vi "GOOP_TcpIpListener.vi"() -> ()   [LabVIEW 2020]
uses:
  <resource>/Framework/Providers/Open_GDS/SubVIs/GOOP_UMLEditor_CallMainAction.ctl
panel:
  out "error out":errorcluster
  out "Numeric 2":u32
  out "remote port":u16
  out "remote address":string
  out "Numeric":i32
  out "data out":string
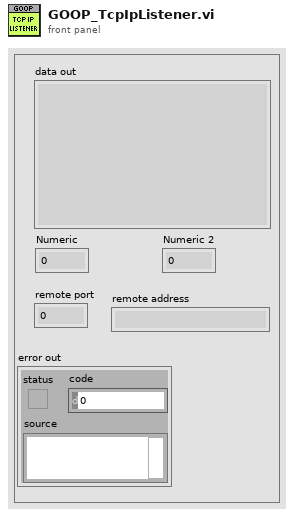
[diagram p1: front panel]
types:
  T1 = enum32{"invalid OS target", "Mac OS", "Windows 3.1", "Windows 95/NT", "Solaris 1", "Solaris 2", "HP-UX", "PowerMAX", "Linux", "Irix", "Rhapsody", "BeOS", "AIX", "OSF1", "VxWorks", "PharLap", "Carbon", "RTX", "Windows x64", "Linux x64"}
  T2 = enum32{"invalid OS target", "Mac OS", "Windows 3.1", "Windows 95/NT", "Solaris 1", "Solaris 2", "HP-UX", "PowerMAX", "Linux", "Irix", "Rhapsody", "BeOS", "AIX", "OSF1", "VxWorks", "PharLap", "Carbon", "RTX", "Windows x64", "Linux x64", "Mac OS X x64"}
  T3 = enum16{"Standard", "Buffered", "CRLF", "Immediate"}
  T4 = typedef "GOOP_UMLEditor_CallMainAction.ctl" = enum16{"OpenUmlEditor", "ReverseEngineering:WholeProject", "ReverseEngineering:OneClass", "ReverseEngineering:OneVI", "ShowInStateDiagram:OneVI", "OpenUMLFile"}
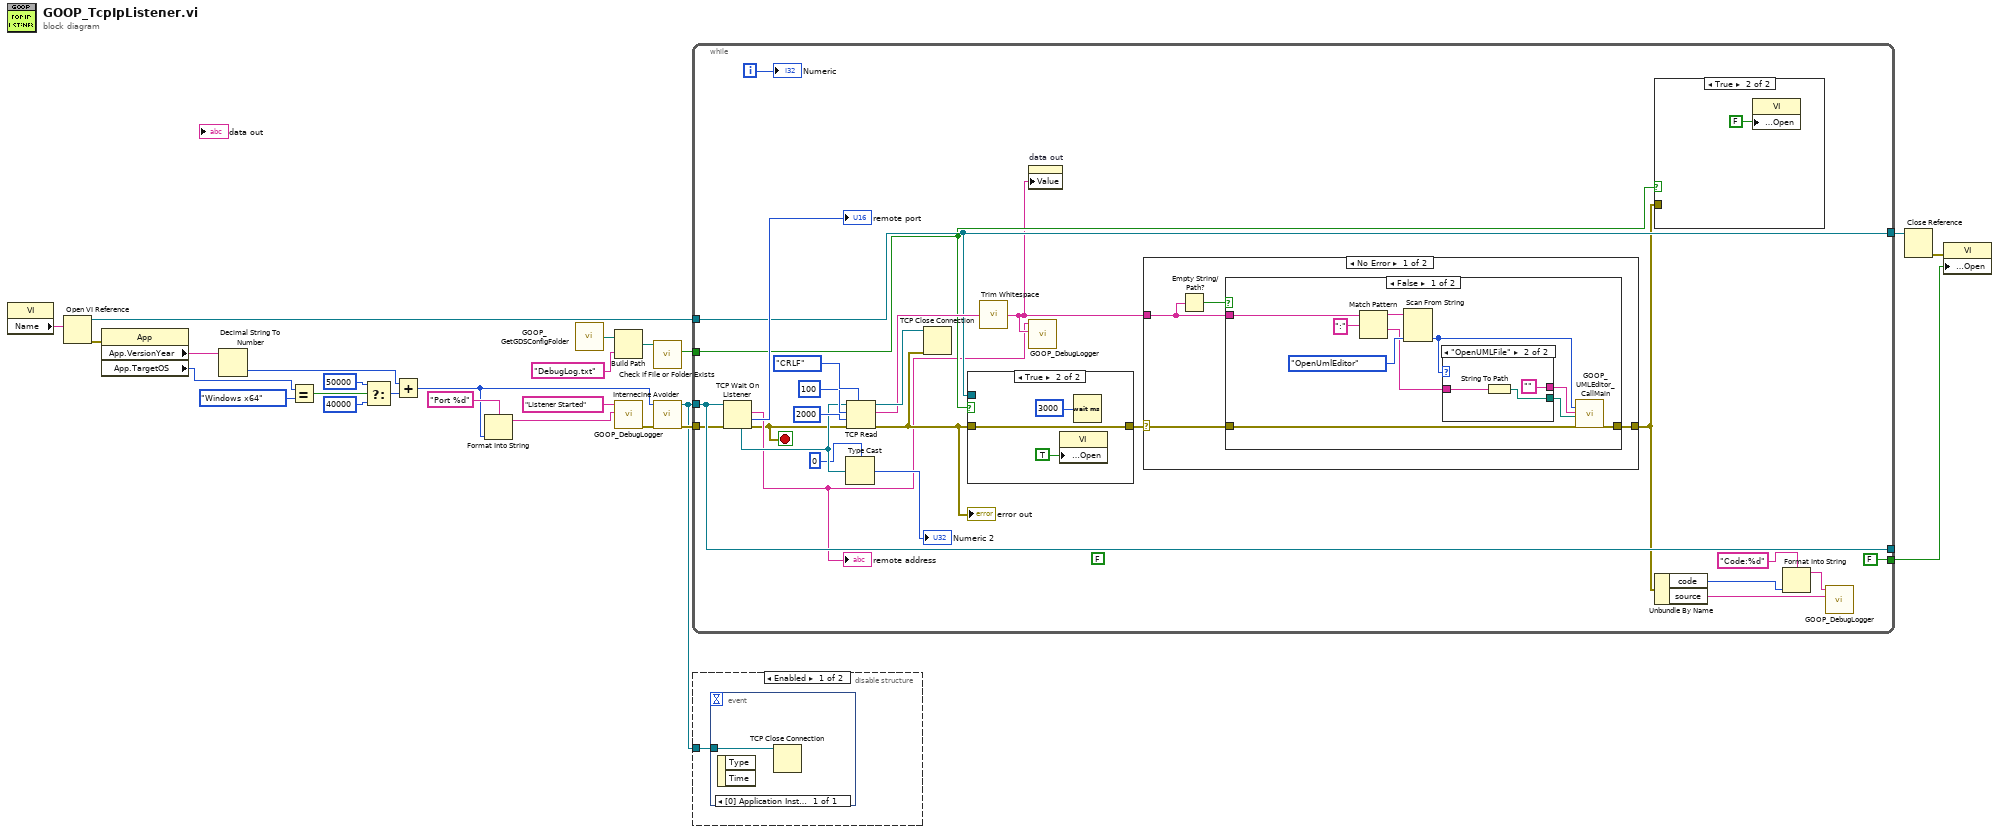
[diagram p0: block diagram]
diagram:
  n1 = property class="VI"() -> ("Name"=w5:string)  [unwired: 2 in, 2 out]
  n2 = Open VI Reference(vi path=w5) -> (vi reference=w6:refnum<vi>, error out=w4:errorcluster)  [unwired: 5 in]
  n3 = property class="App"(error in=w4) -> ("App.VersionYear"=w25:string, "App.TargetOS"=w20:T2)  [unwired: 1 in, 2 out]
  n4 = Decimal String To Number(string=w25) -> (number=w24:i32)  [unwired: 2 in, 1 out]
  n5 = Equal?(x=w20, y=T1."Windows x64") -> (x = y?=w18:bool)
  n6 = Select(t=50000 ("y"), s=w18, f=40000 ("y")) -> (s? t:f=w15:i32)
  n7 = Add(x=w24, y=w15) -> (x+y=w11:i32)
  n8 = Format Into String(format string="Port %d", w11) -> (resulting string=w10:string)  [unwired: 2 in, 1 out]
  n9 = call <resource>:"GOOP_GetGDSConfigFolder.vi"() -> ("GDSFolderPath"=w2:path)
  n10 = Build Path(base path=w2, name or relative path="DebugLog.txt") -> (appended path=w1:path)
  n11 = call <resource>:"GOOP_DebugLogger.vi"("Data"=w10, "State"="Listener Started") -> ("error out"=w8:errorcluster)  [unwired: 7 in, 2 out]
  n12 = call <vilib>:"Check if File or Folder Exists.vi"("path"=w1) -> ("file or folder exists?"=w14:bool)  [unwired: 8 in, 2 out]
  n13 = call <vilib>:"Internecine Avoider.vi"("error in"=w8, "port"=w11) -> ("error out"=w21:errorcluster, "connection ID"=w7:refnum<k5>)  [unwired: 2 in, 6 out]
  n14 = while {
    tunnel: [w45] -> _
    tunnel: [FALSE ("Wait Until Done")] -> w23
    tunnel: w6 -> [w37]
    tunnel: [w37] -> w22
    tunnel: w7 -> [w45]
    tunnel: w21 -> [w44]
    tunnel: w14 -> [w36]
    i -> [w39]
    stop <- w26 stop-if-true
    (unwired) FALSE ("Front Panel Window:Open")
    n15 = TCP Wait On Listener(8:w44, 11:w45) -> (0:w26:errorcluster, 1:→"remote port":u16, 2:w32:string, 4:w41:refnum<k5>)  [unwired: 2 in, 1 out]
    "remote address" <- w32
    n16 = Type Cast(type=u32 0 ("Numeric 2"), x=w41) -> (*(type *) &x=→"Numeric 2":u32)
    n17 = TCP Read(connection ID=w41, bytes to read=100, error in (no error)=w26, 7:T3."CRLF" ("mode (standard)"), 9:2000 ("timeout ms (25000)")) -> (connection ID out=w47:refnum<k5>, data out=w43:string, error out=w34:errorcluster)
    "error out" <- w34
    n18 = TCP Close Connection(connection ID=w47, error in (no error)=w34) -> ()  [unwired: 1 in, 2 out]
    n19 = case shown="True" w36 {
      tunnel: w37 -> [_ _]
      tunnel: w34 -> [w52 w54]
      tunnel: [w52 w54] -> w35
      frame False {
      }
      frame True {
        n20 = property class="VI"("Front Panel.Open"=TRUE ("Front Panel Window:Open")) -> ()  [unwired: 2 in, 2 out]
        n21 = Wait (ms)(milliseconds to wait=u32 3000) -> ()  [unwired: 1 out]
      }
    }
    n22 = call <vilib>:"Trim Whitespace.vi"("string"=w43) -> ("trimmed string"=w33:string)  [unwired: 1 in]
    n23 = property on="data out" class="Str"("Value"=w33) -> ()  [unwired: 2 in, 2 out]
    n24 = call <resource>:"GOOP_DebugLogger.vi"("Data"=w33, "State"=w32) -> ()  [unwired: 7 in, 3 out]
    n25 = case shown="No Error" w35 {
      selector: w35 -> [w59 w74]
      tunnel: w33 -> [w57 _]
      tunnel: [w58 w74] -> w31
      frame No Error {
        n26 = Empty String/Path?(string/path=w57) -> (empty?=w56:bool)
        n27 = case shown="False" w56 {
          tunnel: w57 -> [w68 _]
          tunnel: w59 -> [w62 w73]
          tunnel: [w61 w73] -> w58
          frame False {
            n28 = Match Pattern(string=w68, regular expression=":") -> (before substring=w60:string, after substring=w64:string)  [unwired: 3 out]
            n29 = Scan From String(input string=w60, default 1=GOOP_UMLEditor_CallMainAction."OpenUmlEditor" ("Enum")) -> (output 1=w66:T4)  [unwired: 3 in, 3 out]
            n30 = case shown="\"OpenUMLFile\"" w66 {
              tunnel: [_ ""] -> w65
              tunnel: w64 -> [_ w72]
              tunnel: [_ w71] -> w63
              frame "OpenUmlEditor", Default {
              }
              frame "OpenUMLFile" {
                n31 = String To Path(string=w72) -> (path=w71:path)
              }
            }
            n32 = call <resource>:"GOOP_UMLEditor_CallMain.vi"("Enum"=w66, "Project"=w65, "Class/VI-Path"=w63, "error in (no error)"=w62) -> ("error out"=w61:errorcluster)  [unwired: 15 in]
          }
          frame True {
          }
        }
      }
      frame Error {
      }
    }
    n33 = case shown="True" w36 {
      tunnel: w31 -> [_ _]
      frame False {
      }
      frame True {
        n34 = property class="VI"("Front Panel.Open"=FALSE ("Front Panel Window:Open")) -> ()  [unwired: 2 in, 2 out]
      }
    }
    n35 = Unbundle By Name(w31) -> ("code"=w28:i32, "source"=w30:string)
    n36 = Format Into String(format string="Code:%d", w28) -> (resulting string=w29:string)  [unwired: 2 in, 1 out]
    n37 = call <resource>:"GOOP_DebugLogger.vi"("Data"=w30, "State"=w29) -> ()  [unwired: 7 in, 3 out]
    "Numeric" <- w39
  }
  n38 = disable-structure shown="Enabled" {
    disable-tunnel: w7 -> [w75 _]
    frame Enabled {
      n39 = event shown="[0] Application Instance Close" {
        selector: _ -> [_]
        dyn-events: _ -> [_]
        timeout: _ -> [_]
        tunnel: w75 -> [w76]
        event Application Instance Close {
          n40 = event-data() -> ()  [unwired: 1 in, 2 out]
          n41 = TCP Close Connection(connection ID=w76) -> ()  [unwired: 2 in, 2 out]
        }
      }
    }
    frame Disabled {
    }
  }
  n42 = Close Reference(reference=w22) -> (error out=w9:errorcluster)  [unwired: 1 in]
  n43 = property class="VI"(error in=w9, "Front Panel.Open"=w23) -> ()  [unwired: 1 in, 2 out]
